vi "BlinkinLights.vi"(0 "Basestrip Red":T1, 1 "Basestrip Green":T1, 2 "Basestrip Blue":T1, 3 "Liftstrip Red":T1, 4 "Liftstrip Green":T1, 5 "Liftstrip Blue":T1, 7 "Licenseplate Blue":T1, 9 "Licenseplate Red":T1) -> ()   [LabVIEW 2015]
doc: "BlinkinLights will turn all the lights on or off based on the Light intensity values. Currently only values of 0 or 1 (on or off) are supported (as of 1-31-15). Values are taken from RobotValues global variable and the ports of the vi's must given from another vi."
uses:
  <vilib>/Rock Robotics/WPI/PWM/WPI_PWMDeviceRef.ctl
  <vilib>/Rock Robotics/SystemInterfaces/DIO/FPGA_DIOPWMChannel.ctl
  Robot Values.vi
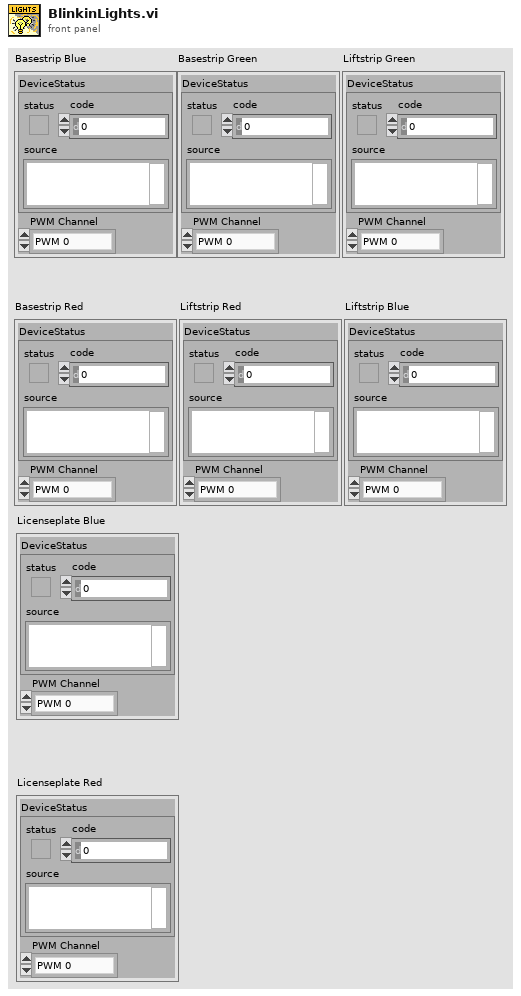
[diagram p1: front panel]
types:
  T1 = typedef "WPI_PWMDeviceRef.ctl" = cluster{"DeviceStatus":errorcluster, "PWM Channel":T2}
  T2 = typedef "FPGA_DIOPWMChannel.ctl" = enum8{"PWM 0", "PWM 1", "PWM 2", "PWM 3", "PWM 4", "PWM 5", "PWM 6", "PWM 7", "PWM 8", "PWM 9", "PWM MXP 0", "PWM MXP 1", "PWM MXP 2", "PWM MXP 3", "PWM MXP 4", "PWM MXP 5", "PWM MXP 6", "PWM MXP 7", "PWM MXP 8", "PWM MXP 9", "Invalid"}
  T3 = cluster{"Light level Base":dbl[], "Light level Lift":dbl[], "Light Level License plates":dbl[]}
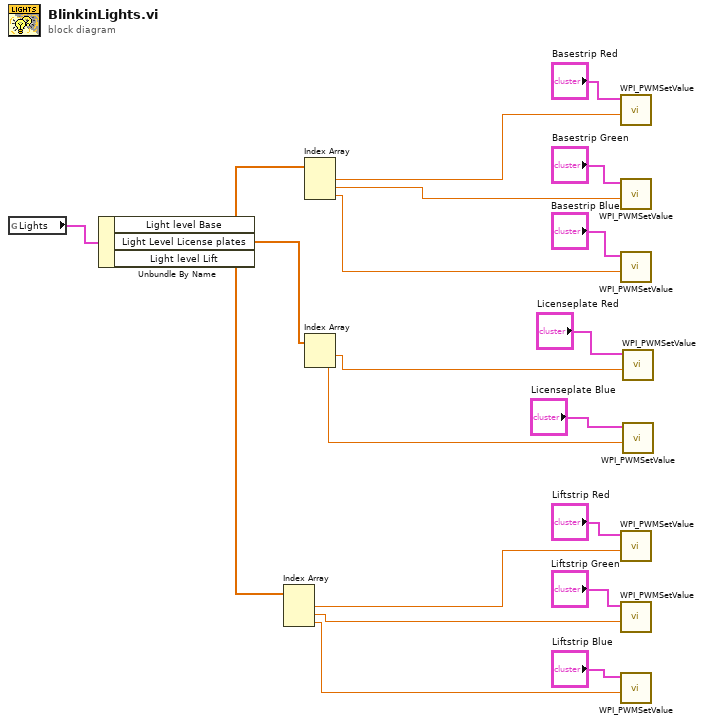
[diagram p0: block diagram]
diagram:
  n1 = global read "Robot Values.vi" "Lights"() -> (w14:T3)
  n2 = Unbundle By Name(w14) -> ("Light level Base"=w12:dbl[], "Light Level License plates"=w5:dbl[], "Light level Lift"=w13:dbl[])
  n3 = Index Array(array=w13) -> (element #1=w8:dbl, element #2=w7:dbl, element #3=w6:dbl)  [unwired: 3 in]
  n4 = Index Array(array=w12) -> (element #1=w11:dbl, element #2=w10:dbl, element #3=w9:dbl)  [unwired: 3 in]
  n5 = Index Array(array=w5) -> (element #1=w4:dbl, element #2=w3:dbl)  [unwired: 2 in]
  n6 = call <vilib>:"WPI_PWMSetValue.vi"("Value"=w11, "PWMDeviceRef"="Basestrip Red") -> ()  [unwired: 8 in, 2 out]
  n7 = call <vilib>:"WPI_PWMSetValue.vi"("Value"=w10, "PWMDeviceRef"="Basestrip Green") -> ()  [unwired: 8 in, 2 out]
  n8 = call <vilib>:"WPI_PWMSetValue.vi"("Value"=w9, "PWMDeviceRef"="Basestrip Blue") -> ()  [unwired: 8 in, 2 out]
  n9 = call <vilib>:"WPI_PWMSetValue.vi"("Value"=w8, "PWMDeviceRef"="Liftstrip Red") -> ()  [unwired: 8 in, 2 out]
  n10 = call <vilib>:"WPI_PWMSetValue.vi"("Value"=w7, "PWMDeviceRef"="Liftstrip Green") -> ()  [unwired: 8 in, 2 out]
  n11 = call <vilib>:"WPI_PWMSetValue.vi"("Value"=w6, "PWMDeviceRef"="Liftstrip Blue") -> ()  [unwired: 8 in, 2 out]
  n12 = call <vilib>:"WPI_PWMSetValue.vi"("Value"=w4, "PWMDeviceRef"="Licenseplate Red") -> ()  [unwired: 8 in, 2 out]
  n13 = call <vilib>:"WPI_PWMSetValue.vi"("Value"=w3, "PWMDeviceRef"="Licenseplate Blue") -> ()  [unwired: 8 in, 2 out]
